vi "Customizing Shortcut Menus.vi"() -> ()   [LabVIEW 2014]
doc: "该范例演示了创建自定义运行时快捷菜单的方法。运行时快捷菜单可在输入控件和显示控件上静态或动态配置。"
panel:
  out "波形图":dbl[][](graph)
  out "已选数据集":dbl[](array[numeric]) format="%#_4g"
  out "全部测试结果":dbl[][](array[numeric]) format="%#_4g"
  in  "运行测试":bool
  in  "停止":bool
  in  "测试列表":i32(listbox)=-1
  # "概述：演示使用菜单函数在前面板对象上创建动态运行时快捷菜单，并响应这些对象上的菜单选择。\n操作步骤：\n1. 运行VI。\n2. 多次单击运行测试按钮。\n3. 右键单击测试列表列表框并尝试使用一些运行时快捷菜单选项。\n4. 右键单击全部测试结果数组并选择“绘制全部数据”，在波形图中绘制全部数据。\n5. 单击停止可停止VI。"
  # "注：全部测试结果数组使用静态快捷菜单。关于配置静态自定义运行时快捷菜单的详细信息，见程序框图。"
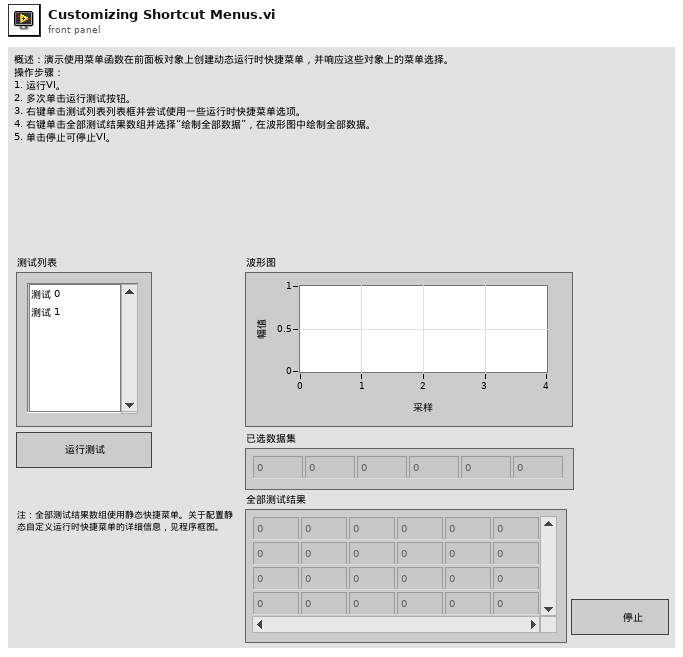
[diagram p1: front panel]
types:
  T1 = typedef "LVPoint32TypeDef.ctl" = cluster{"Horizontal":i32, "Vertical":i32}
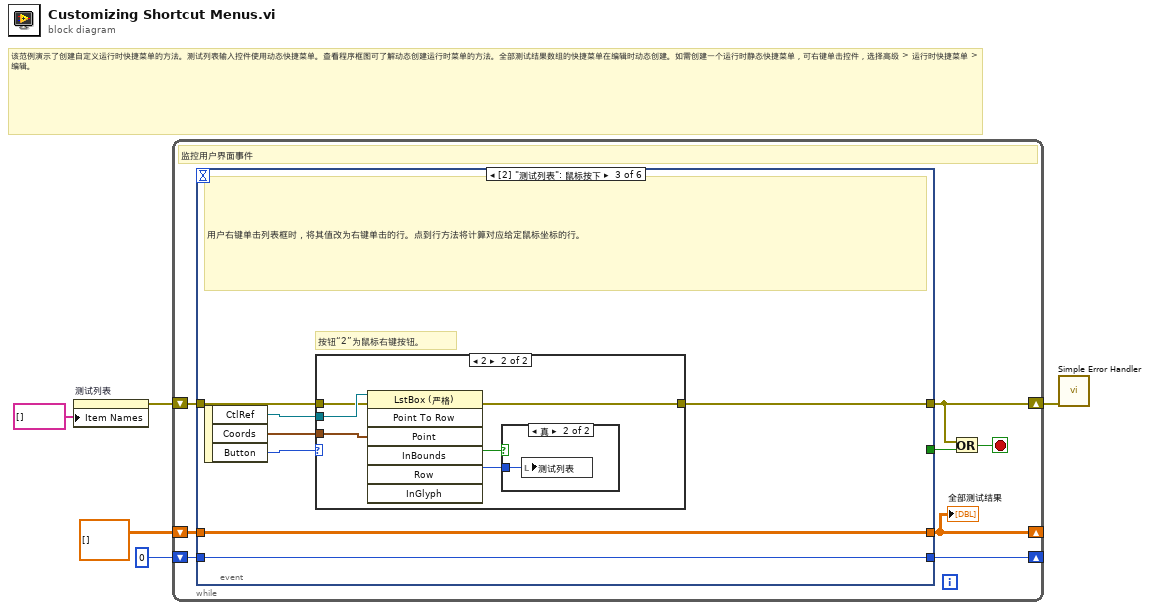
[diagram p0: block diagram]
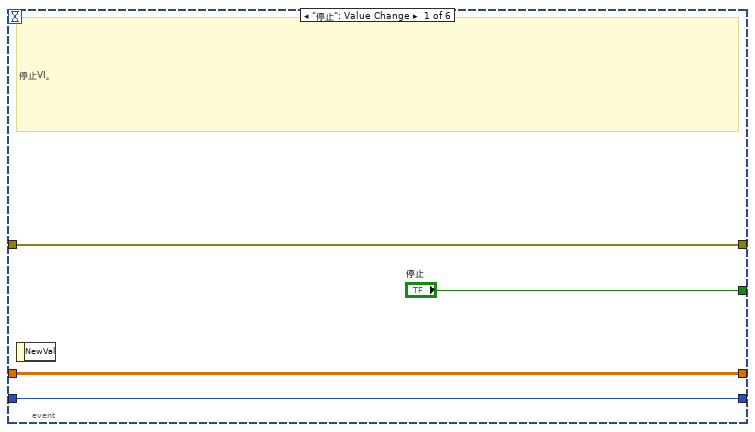
[diagram p2: hidden frame]
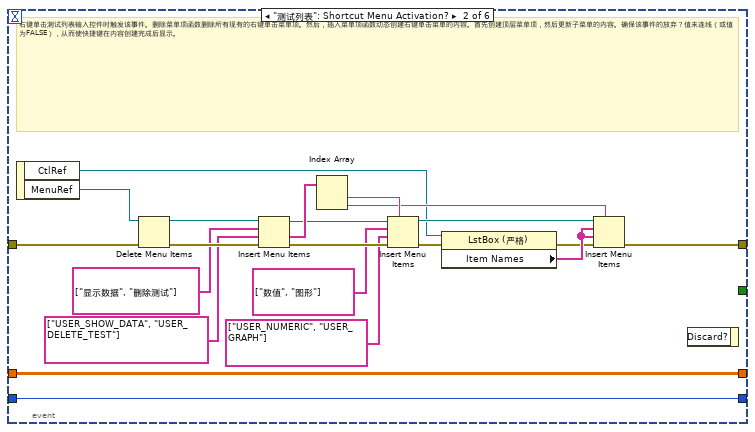
[diagram p3: hidden frame]
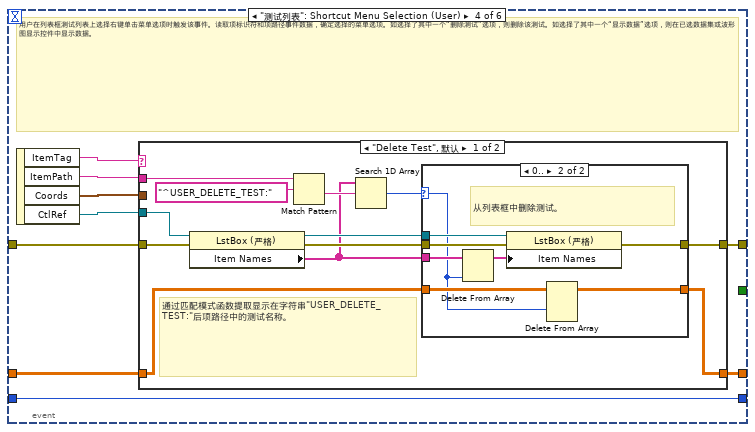
[diagram p6: hidden frame]
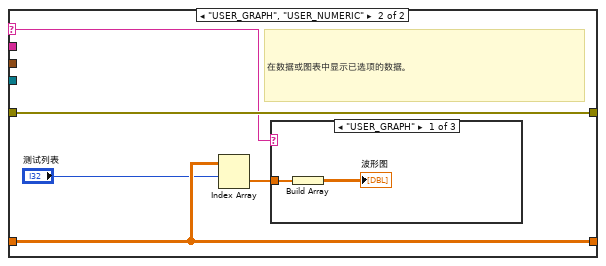
[diagram p8: hidden frame]
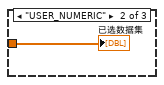
[diagram p9: hidden frame]
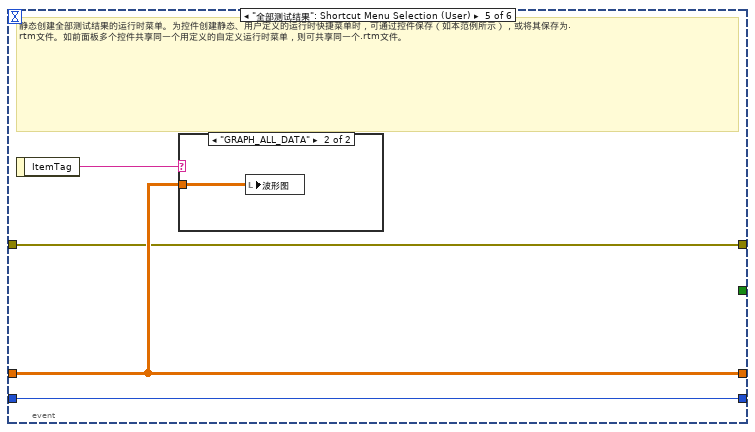
[diagram p11: hidden frame]
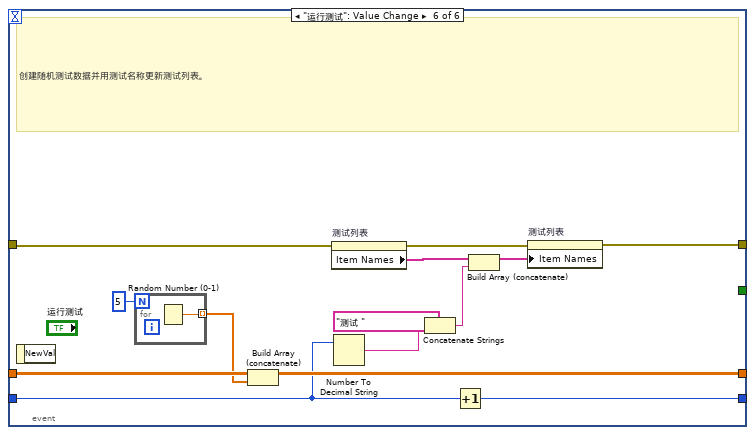
[diagram p13: hidden frame]
diagram:
  # "该范例演示了创建自定义运行时快捷菜单的方法。测试列表输入控件使用动态快捷菜单。查看程序框图可了解动态创建运行时菜单的方法。全部测试结果数组的快捷菜单在编辑时动态创建。如需创建一个运行时静态快捷菜单，可右键单击控件，选择高级 > 运行时快捷菜单 > 编辑。"
  n1 = property on="测试列表" class="LstBox (严格)"("Item Names"=string[] []) -> (error out=w3:errorcluster)  [unwired: 2 in, 1 out]
  n2 = while {
    shift-right: [w9] -> _
    shift-left: dbl[][] [] -> [w12]
    shift-right: [w10] -> _
    shift-left: 0 -> [w11]
    shift-right: [w6] -> w1
    shift-left: w3 -> [w8]
    stop <- w7 stop-if-true
    # "监控用户界面事件"
    n3 = event shown="[2] \"测试列表\": 鼠标按下" {
      selector: _ -> [_ _ _ _ _ _]
      dyn-events: _ -> [_ _ _ _ _ _]
      timeout: _ -> [_ _ _ _ _ _]
      tunnel: ["停止" _ _ _ _ _] -> w13
      tunnel: w12 -> [w16 w33 w43 w60 w95 w110]
      tunnel: [w16 w33 w43 w58 w95 w108] -> w9
      tunnel: w11 -> [w15 w23 w42 w57 w96 w101]
      tunnel: [w15 w23 w42 w57 w96 w102] -> w10
      tunnel: w8 -> [w14 w22 w40 w56 w93 w99]
      tunnel: [w14 w21 w39 w55 w93 w98] -> w6
      event "停止": Value Change {
        # "停止VI。"
        n4 = event-data() -> ()  [unwired: 1 in, 1 out]
      }
      event "测试列表": Shortcut Menu Activation? {
        # "右键单击测试列表输入控件时触发该事件。删除菜单项函数删除所有现有的右键单击菜单项。然后，插入菜单项函数动态创建右键单击菜单的内容。首先创建顶层菜单项，然后更新子菜单的内容。确保该事件的放弃？值未连线（或值为FALSE），从而使快捷键在内容创建完成后显示。"
        n5 = event-data() -> ("CtlRef"=w18:refnum<vi>, "MenuRef"=w38:refnum<k9>)  [unwired: 1 in]
        n6 = Delete Menu Items(6:w22, 9:w38) -> (0:w36:errorcluster, 3:w37:refnum<k9>)  [unwired: 2 in]
        n7 = Insert Menu Items(6:w36, 7:string[] ["USER_SHOW_DATA", "USER_DELETE_TEST"], 8:string[] ["显示数据", "删除测试"] ("L10n_Parent Menus"), 9:w37) -> (0:w30:errorcluster, 1:w32:string[], 3:w29:refnum<k9>)  [unwired: 2 in]
        n8 = Index Array(array=w32) -> (element #1=w31:string, element #2=w25:string)  [unwired: 2 in]
        n9 = Insert Menu Items(5:w31, 6:w30, 7:string[] ["USER_NUMERIC", "USER_GRAPH"] ("item tags"), 8:string[] ["数值", "图形"] ("L10n_Item Names"), 9:w29) -> (0:w20:errorcluster, 3:w26:refnum<k9>)  [unwired: 1 in, 1 out]
        n10 = property class="LstBox (严格)"(reference=w18, error in=w20) -> (error out=w19:errorcluster, "Item Names"=w24:string[])  [unwired: 1 out]
        n11 = Insert Menu Items(5:w25, 6:w19, 7:w24, 8:w24, 9:w26) -> (0:w21:errorcluster)  [unwired: 1 in, 2 out]
        n12 = event-data() -> ()  [unwired: 2 in, 1 out]
      }
      event "测试列表": Mouse Down {
        # "按钮“2”为鼠标右键按钮。"
        # "用户右键单击列表框时，将其值改为右键单击的行。点到行方法将计算对应给定鼠标坐标的行。"
        n13 = event-data() -> ("CtlRef"=w44:refnum<vi>, "Coords"=w45:T1, "Button"=w41:u16)  [unwired: 1 in]
        n14 = case shown="2" w41 {
          tunnel: w45 -> [_ w52]
          tunnel: w44 -> [_ w51]
          tunnel: w40 -> [w46 w49]
          tunnel: [w46 w50] -> w39
          frame Default {
          }
          frame 2 {
            n15 = invoke class="LstBox (严格)" method="Point To Row"(reference=w51, error in=w49, "Point"=w52) -> (error out=w50:errorcluster, "InBounds"=w47:bool, "Row"=w48:i32)  [unwired: 4 in, 4 out]
            n16 = case shown="真" w47 {
              tunnel: w48 -> [_ w53]
              frame False {
              }
              frame True {
                n17 = local write "测试列表"(w53) -> ()
              }
            }
          }
        }
      }
      event "测试列表": Shortcut Menu Selection (User) {
        # "用户在列表框测试列表上选择右键单击菜单选项时触发该事件。读取项标识符和项路径事件数据，确定选择的菜单选项。如选择了其中一个“删除测试”选项，则删除该测试。如选择了其中一个“显示数据”选项，则在已选数据集或波形图显示控件中显示数据。"
        n18 = event-data() -> ("ItemTag"=w62:string, "ItemPath"=w61:string, "Coords"=w59:T1, "CtlRef"=w54:refnum<vi>)  [unwired: 1 in]
        n19 = case shown="\"Delete Test\", 默认" w62 {
          selector: w62 -> [_ w86]
          tunnel: w61 -> [w74 _]
          tunnel: w54 -> [w72 _]
          tunnel: w60 -> [w67 w88]
          tunnel: w59 -> [_ _]
          tunnel: [w66 w88] -> w58
          tunnel: w56 -> [w65 w87]
          tunnel: [w64 w87] -> w55
          frame "Delete Test", Default {
            # "通过匹配模式函数提取显示在字符串\"USER_DELETE_TEST:\"后项路径中的测试名称。"
            n20 = property class="LstBox (严格)"(reference=w72, error in=w65) -> (reference out=w70:refnum<vi>, error out=w69:errorcluster, "Item Names"=w68:string[])
            n21 = Match Pattern(string=w74, regular expression="^USER_DELETE_TEST:") -> (after substring=w71:string)  [unwired: 1 in, 3 out]
            n22 = Search 1D Array(1D array=w68, element=w71) -> (index of element=w63:i32)  [unwired: 1 in]
            n23 = case shown="0.." w63 {
              selector: w63 -> [_ w77]
              tunnel: w70 -> [_ w84]
              tunnel: w69 -> [w75 w83]
              tunnel: w68 -> [_ w82]
              tunnel: w67 -> [w76 w80]
              tunnel: [w76 w79] -> w66
              tunnel: [w75 w78] -> w64
              frame Default {
              }
              frame 0.. {
                # "从列表框中删除测试。"
                n24 = Delete From Array(array=w82, index=w77) -> (array with subset deleted=w81:string[])  [unwired: 1 in, 1 out]
                n25 = property class="LstBox (严格)"(reference=w84, error in=w83, "Item Names"=w81) -> (error out=w78:errorcluster)  [unwired: 1 out]
                n26 = Delete From Array(array=w80, index (row)=w77) -> (array with subset deleted=w79:dbl[][])  [unwired: 2 in, 1 out]
              }
            }
          }
          frame "USER_GRAPH", "USER_NUMERIC" {
            # "在数据或图表中显示已选项的数据。"
            n27 = Index Array(array=w88, index (row)="测试列表") -> (element=w89:dbl[])  [unwired: 1 in]
            n28 = case shown="\"USER_GRAPH\"" w86 {
              tunnel: w89 -> [w90 w92 _]
              frame "USER_GRAPH" {
                n29 = Build Array(w90) -> (→"波形图":dbl[][])
              }
              frame "USER_NUMERIC" {
                "已选数据集" <- w92
              }
              frame Default {
              }
            }
          }
        }
      }
      event "全部测试结果": Shortcut Menu Selection (User) {
        # "静态创建全部测试结果的运行时菜单。为控件创建静态、用户定义的运行时快捷菜单时，可通过控件保存（如本范例所示），或将其保存为.rtm文件。如前面板多个控件共享同一个用定义的自定义运行时菜单，则可共享同一个.rtm文件。"
        n30 = event-data() -> ("ItemTag"=w94:string)  [unwired: 1 in]
        n31 = case shown="\"GRAPH_ALL_DATA\"" w94 {
          tunnel: w95 -> [_ w97]
          frame Default {
          }
          frame "GRAPH_ALL_DATA" {
            n32 = local write "波形图"(w97) -> ()
          }
        }
      }
      event "运行测试": Value Change {
        # "创建随机测试数据并用测试名称更新测试列表。"
        n33 = event-data() -> ()  [unwired: 1 in, 1 out]
        n34 = for {
          N: 5 -> [_]
          tunnel: [w112] -> w109 mode=indexing
          n35 = Random Number (0-1)() -> (number: 0 to 1=w112:dbl)
        }
        n36 = Build Array (concatenate)(w110, w109) -> (w108:dbl[][])
        n37 = property on="测试列表" class="LstBox (严格)"(error in=w99) -> (error out=w107:errorcluster, "Item Names"=w106:string[])  [unwired: 1 in, 1 out]
        n38 = Number To Decimal String(number=w101) -> (decimal integer string=w100:string)  [unwired: 1 in]
        n39 = Concatenate Strings("测试 " ("L10n_Test"), w100) -> (w103:string)
        n40 = Increment(x=w101) -> (x+1=w102:i32)
        n41 = Build Array (concatenate)(w106, w103) -> (w105:string[])
        n42 = property on="测试列表" class="LstBox (严格)"(error in=w107, "Item Names"=w105) -> (error out=w98:errorcluster)  [unwired: 1 in, 1 out]
      }
    }
    "全部测试结果" <- w9
    n43 = Or(x=w6, y=w13) -> (x .or. y?=w7:bool)
  }
  n44 = call <vilib>:"Simple Error Handler.vi"("error in (no error)"=w1) -> ()  [unwired: 4 in, 5 out]
